vi "Abre_prioridade_file_client.vi"(11 "Meu_Ip":string) -> (0 "error out":errorcluster, 3 "refnum":T1)   [LabVIEW 2019]
uses:
  <vilib>/Utility/config.llb/Config Data RefNum.ctl
  <vilib>/Utility/config.llb/NI_LVConfig.lvlib
panel:
  out "appended path":path
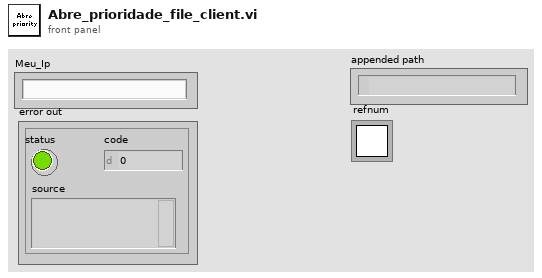
[diagram p1: front panel]
types:
  T1 = typedef "NI_LVConfig.lvlib/Config Data RefNum.ctl" = refnum<k1>
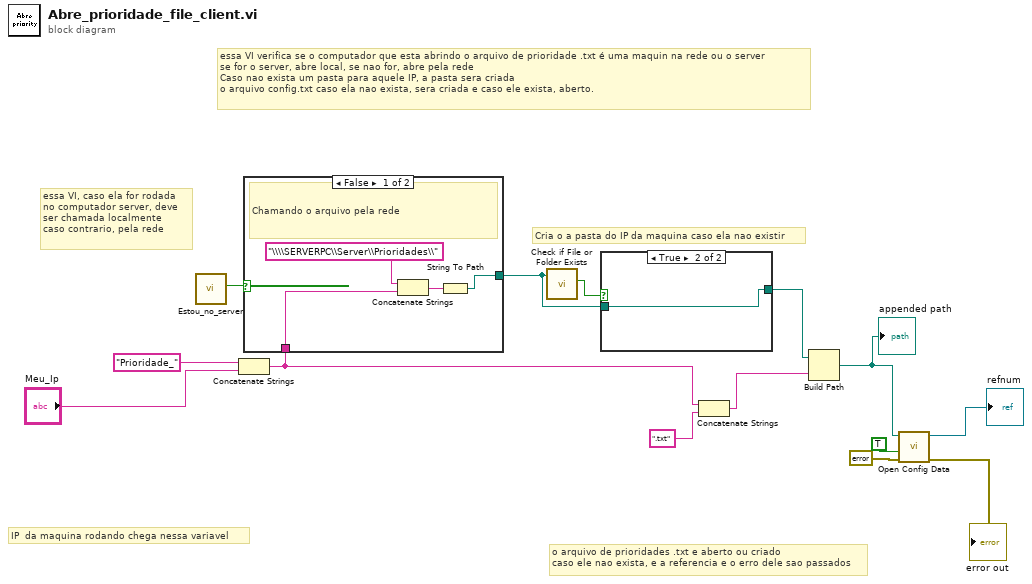
[diagram p0: block diagram]
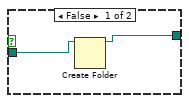
[diagram p2: hidden frame]
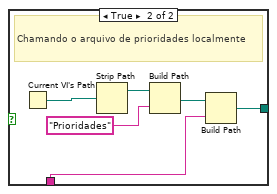
[diagram p3: hidden frame]
diagram:
  # "essa VI verifica se o computador que esta abrindo o arquivo de prioridade .txt é uma maquin na rede ou o server\nse for o server, abre local, se nao for, abre pela rede\nCaso nao exista um pasta para aquele IP, a pasta sera criada\no arquivo config.txt caso ela nao exista, sera criada e caso ele exista, aberto."
  # "o arquivo de prioridades .txt e aberto ou criado\ncaso ele nao exista, e a referencia e o erro dele sao passados"
  # "Cria o a pasta do IP da maquina caso ela nao existir"
  # "essa VI, caso ela for rodada\nno computador server, deve\nser chamada localmente\ncaso contrario, pela rede"
  # "IP  da maquina rodando chega nessa variavel"
  n1 = call "Estou_no_server.vi"() -> ("Estou no serve?"=w9:bool)  [unwired: 11 in]
  n2 = Concatenate Strings("Prioridade_" ("string"), "Meu_Ip") -> (w3:string)
  n3 = case shown="False" w9 {
    tunnel: w3 -> [w17 w20]
    tunnel: [w15 w19] -> w6
    frame False {
      # "Chamando o arquivo pela rede"
      n4 = Concatenate Strings("\\\\SERVERPC\\Server\\Prioridades\\", w17) -> (w16:string)
      n5 = String To Path(string=w16) -> (path=w15:path)
    }
    frame True {
      # "Chamando o arquivo de prioridades localmente"
      n6 = Current VI's Path() -> (path=w23:path)
      n7 = Strip Path(path=w23) -> (stripped path=w24:path)  [unwired: 1 out]
      n8 = Build Path(base path=w24, name or relative path="Prioridades") -> (appended path=w21:path)
      n9 = Build Path(base path=w21, name or relative path=w20) -> (appended path=w19:path)
    }
  }
  n10 = call <vilib>:"Check if File or Folder Exists.vi"("path"=w6) -> ("file or folder exists?"=w7:bool)  [unwired: 8 in, 2 out]
  n11 = case shown="True" w7 {
    tunnel: w6 -> [w26 w27]
    tunnel: [w25 w27] -> w5
    frame False {
      n12 = Create Folder(path (use dialog)=w26) -> (created path=w25:path)  [unwired: 2 in, 2 out]
    }
    frame True {
    }
  }
  n13 = Concatenate Strings(w3, ".txt") -> (w2:string)
  n14 = Build Path(base path=w5, name or relative path=w2) -> (appended path=w1:path)
  "appended path" <- w1
  n15 = call <vilib>:"Open Config Data.vi"("error in (no error)"=errorcluster {"status"=FALSE, "code"=0, "source"=""}, "create file if necessary (T)"=TRUE, "configuration file path"=w1) -> ("error out"=→"error out":errorcluster, "refnum"=→"refnum":T1)  [unwired: 6 in, 1 out]
